vi "Filter Control Drag Starting Event.vi"(8 "error in (no error)":errorcluster, 10 "ControlDragStartingMsg":refnum<class "ControlDragStartingMsg.lvclass">, 11 "File Explorer Event Filter in":refnum<class "File Explorer Event Filter.lvclass">) -> (0 "error out":errorcluster, 1 "Discard?":bool, 2 "Filtered Event Data":T1, 3 "File Explorer Event Filter out":refnum<class "File Explorer Event Filter.lvclass">, 5 "Data Filtered?":bool)   [LabVIEW 2019, in "File Explorer.lvlib" / "File Explorer Event Filter.lvclass"]
uses:
  <vilib>/gpm_packages/@cs/file-explorer-extension/Source/File Explorer/File Explorer Event Filter/File Explorer Event Filter.lvclass
  <vilib>/gpm_packages/@cs/mva-viewable/Source/ActorEvents/IEventAggregator Messages/ControlDragStartingMsg/ControlDragStartingMsg.lvclass
  <vilib>/gpm_packages/@cs/file-explorer-extension/Source/File Explorer/File Explorer Event Filter/File Explorer Event Filter.lvclass/File Explorer Event Filter.ctl
  <vilib>/gpm_packages/@cs/file-explorer-extension/Source/File Explorer/File Explorer Messages/Handle Drag Starting Msg/Handle Drag Starting Msg.lvclass/Handle Drag Starting Msg.ctl
  <vilib>/gpm_packages/@cs/mva-viewable/Source/ActorEvents/IEventAggregator Messages/ControlDragStartingMsg/ControlDragStartingMsg.lvclass/ControlDragStartingMsg.ctl
  <vilib>/gpm_packages/@cs/file-explorer-extension/Source/Application Dependencies/Application Types/Drag Starting Filtered Event Data.ctl
  <vilib>/gpm_packages/@cs/actor-framework-messages/Source/RoundTripMessage/RoundTripMessage.lvclass/RoundTripMessage.ctl
  <vilib>/ActorFramework/Message Enqueuer/Message Enqueuer.lvclass/Message Enqueuer.ctl
  <vilib>/ActorFramework/Message Enqueuer/Enqueue.vi
  <vilib>/gpm_packages/@cs/file-explorer-extension/Source/File Explorer/File Explorer Messages/Handle Drag Starting Msg/Handle Drag Starting Msg.lvclass
  C:/Program Files/National Instruments/LabVIEW 2019/vi.lib/gpm_packages/@cs/actor-framework-messages/Source/RoundTripMessage/RoundTripMessage.lvclass
  <vilib>/gpm_packages/@cs/actor-framework-messages/Source/RoundTripMessage/RoundTripMessage.lvclass
  C:/Program Files/National Instruments/LabVIEW 2019/vi.lib/ActorFramework/Message/Message.lvclass
  <vilib>/ActorFramework/Message Priority Queue/Priority Enqueue.vi
  <vilib>/gpm_packages/@cs/file-explorer-extension/Source/File Explorer/File Explorer.lvlib
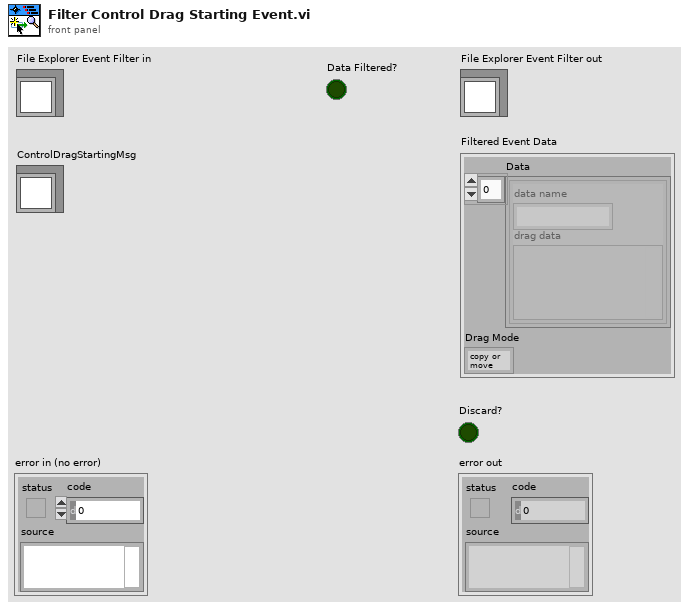
[diagram p1: front panel]
types:
  T1 = cluster{"Data":cluster{"data name":string, "drag data":variant}[], "Drag Mode":enum32{"copy or move", "copy only", "move only"}}
  T2 = typedef "File Explorer.lvlib/Drag Starting Filtered Event Data.ctl" = cluster{"Drag Mode":enum32{"copy or move", "copy only", "move only"}, "Data Filtered?":bool, "Discard?":bool, "Tag":string, "Dragging?":bool}
  T3 = cluster{"data name":string, "drag data":variant}[]
  T4 = cluster{"Shift":bool, "Ctrl":bool, "Alt":bool, "Cmd":bool, "Opt":bool}
  T5 = typedef "LVPoint32TypeDef.ctl" = cluster{"Horizontal":i32, "Vertical":i32}
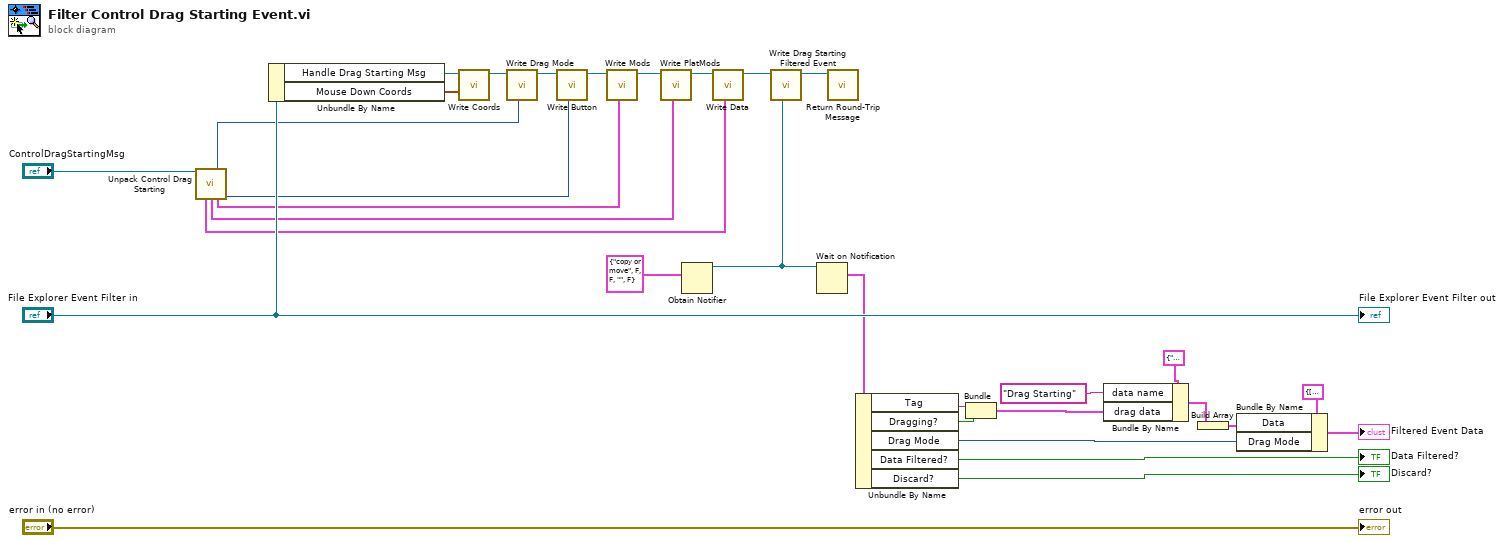
[diagram p0: block diagram]
diagram:
  n1 = call <vilib>:"Unpack Control Drag Starting.vi"("ControlDragStartingMsg In"="ControlDragStartingMsg") -> ("Drag Mode"=w26:enum32{"copy or move", "copy only", "move only"}, "Data"=w18:T3, "PlatMods"=w20:T4, "Mods"=w22:cluster{"Double Click":bool, "Menu Key":bool}, "Button"=w24:u16)  [unwired: 6 in, 4 out]
  n2 = Unbundle By Name("File Explorer Event Filter in") -> ("Handle Drag Starting Msg"=w29:refnum<class "Handle Drag Starting Msg.lvclass">, "Mouse Down Coords"=w28:T5)
  n3 = call <vilib>:"Write Coords.vi"("Coordinates"=w28, "Handle Drag Starting Msg in"=w29) -> ("Handle Drag Starting Msg out"=w27:refnum<class "Handle Drag Starting Msg.lvclass">)  [unwired: 9 in]
  n4 = call <vilib>:"Write Drag Mode.vi"("Drag Mode"=w26, "Handle Drag Starting Msg in"=w27) -> ("Handle Drag Starting Msg out"=w25:refnum<class "Handle Drag Starting Msg.lvclass">)  [unwired: 9 in]
  n5 = call <vilib>:"Write Button.vi"("Button"=w24, "Handle Drag Starting Msg in"=w25) -> ("Handle Drag Starting Msg out"=w23:refnum<class "Handle Drag Starting Msg.lvclass">)  [unwired: 9 in]
  n6 = call <vilib>:"Write Mods.vi"("Mods"=w22, "Handle Drag Starting Msg in"=w23) -> ("Handle Drag Starting Msg out"=w21:refnum<class "Handle Drag Starting Msg.lvclass">)  [unwired: 9 in]
  n7 = call <vilib>:"Write PlatMods.vi"("PlatMods"=w20, "Handle Drag Starting Msg in"=w21) -> ("Handle Drag Starting Msg out"=w19:refnum<class "Handle Drag Starting Msg.lvclass">)  [unwired: 9 in]
  n8 = Obtain Notifier(notification data type=T2 {"Drag Mode"=enum."copy or move", "Data Filtered?"=FALSE, "Discard?"=FALSE, "Tag"="", "Dragging?"=FALSE} ("Drag Starting Filtered Event Data")) -> (notifier out=w16:refnum<notifier>)  [unwired: 3 in, 2 out]
  n9 = call <vilib>:"Write Data.vi"("Data"=w18, "Handle Drag Starting Msg in"=w19) -> ("Handle Drag Starting Msg out"=w17:refnum<class "Handle Drag Starting Msg.lvclass">)  [unwired: 9 in]
  n10 = call <vilib>:"Write Drag Starting Filtered Event.vi"("Drag Starting Filtered Event"=w16, "Handle Drag Starting Msg in"=w17) -> ("Handle Drag Starting Msg out"=w1:refnum<class "Handle Drag Starting Msg.lvclass">)  [unwired: 9 in]
  n11 = Wait on Notification(notifier=w16) -> (notification=w15:T2)  [unwired: 3 in, 3 out]
  n12 = call <vilib>:"Return Round-Trip Message.vi"("RoundTripMessage In"=w1) -> ()  [unwired: 10 in, 1 out]
  n13 = Unbundle By Name(w15) -> ("Tag"=w6:string, "Dragging?"=w5:bool, "Drag Mode"=w4:enum32{"copy or move", "copy only", "move only"}, "Data Filtered?"=→"Data Filtered?":bool, "Discard?"=→"Discard?":bool)
  n14 = Bundle("Tag"=w6, "Dragging?"=w5) -> (w8:cluster{"Tag":string, "Dragging?":bool})  [unwired: 1 in]
  n15 = Bundle By Name(cluster=cluster{"data name":string, "drag data":variant} {"data name"="", "drag data"=variant}, "data name"="Drag Starting", "drag data"=w8) -> (w10:cluster{"data name":string, "drag data":variant})
  n16 = Build Array(w10) -> (w9:T3)
  n17 = Bundle By Name(cluster=T1 {"Data"=[], "Drag Mode"=enum."copy or move"} ("Filtered Event Data"), "Data"=w9, "Drag Mode"=w4) -> (→"Filtered Event Data":T1)
  "error out" <- "error in (no error)"
  "File Explorer Event Filter out" <- "File Explorer Event Filter in"
